vi "Initialize.vi"(8 "error in (no error)":errorcluster, 9 "Enqueuer ID string":string, 10 "Response Msg in":refnum<class "Response Msg.lvclass">, 11 "Response Core in":refnum<class "Response Core.lvclass">) -> (0 "error out":errorcluster, 1 "Wait for Response?":bool, 2 "Response Msg out":refnum<class "Response Msg.lvclass">, 3 "Response Core out":refnum<class "Response Core.lvclass">)   [LabVIEW 2020, in "Publisher.lvlib" / "Response Core.lvclass"]
doc: "Initialize the Response Core\n\nThe default implementation does nothing but return a false in 'Wait for Response?'."
uses:
  Response Core.lvclass
  Response Msg.lvclass
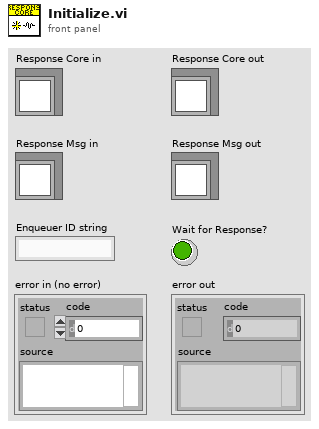
[diagram p1: front panel]
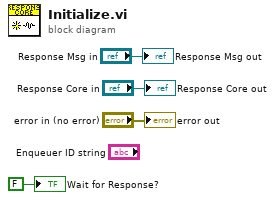
[diagram p0: block diagram]
diagram:
  "error out" <- "error in (no error)"
  "Response Core out" <- "Response Core in"
  "Response Msg out" <- "Response Msg in"
  "Wait for Response?" <- FALSE ("Wait for Response?")
